vi "USRP Sampling.vi"() -> ()   [LabVIEW 2014]
uses:
  <instrlib>/niUSRP/niUSRP Fetch Rx Data (CDB Cluster).vi
panel:
  out "n":i32
  out "output":dbl[][](array[numeric])
  out "Waveform Graph":dbl[](graph)
  out "Iteration":i32
  out "Array":dbl[](array[numeric])
  in  "stop":bool
  in  "Tab Control":enum32{"USRP Setup", "Parameter"}(tab)
  in  "device names":refnum<k15>="192.168.10.2"
  in  "IQ rate":dbl=800000.0 format="%#_6p"
  in  "carrier frequency":dbl=2422000000.0 format="%#_6p"
  in  "gain":dbl=10.0 format="%#_6f"
  out "coerced IQ rate":dbl=800000.0 format="%#_6p"
  out "coerced carrier frequency":dbl=2421999999.997206 format="%#_6p"
  out "coerced gain":dbl=10.0 format="%#_6f"
  out "error out":errorcluster
  in  "active antenna":string="RX2"
  out "Duration(s)":dbl
  in  "Moving\nAverage":bool=TRUE
  in  "Time Window(s)":dbl=0.01 format="%#_6p"
  in  "SamplingTimes":i32=100
  in  "threshold":dbl=1.0
  in  "step":dbl=1.0
  in  "offset":i32
  in  "Method":enum16{"Binary", "Uniform"}(ring)
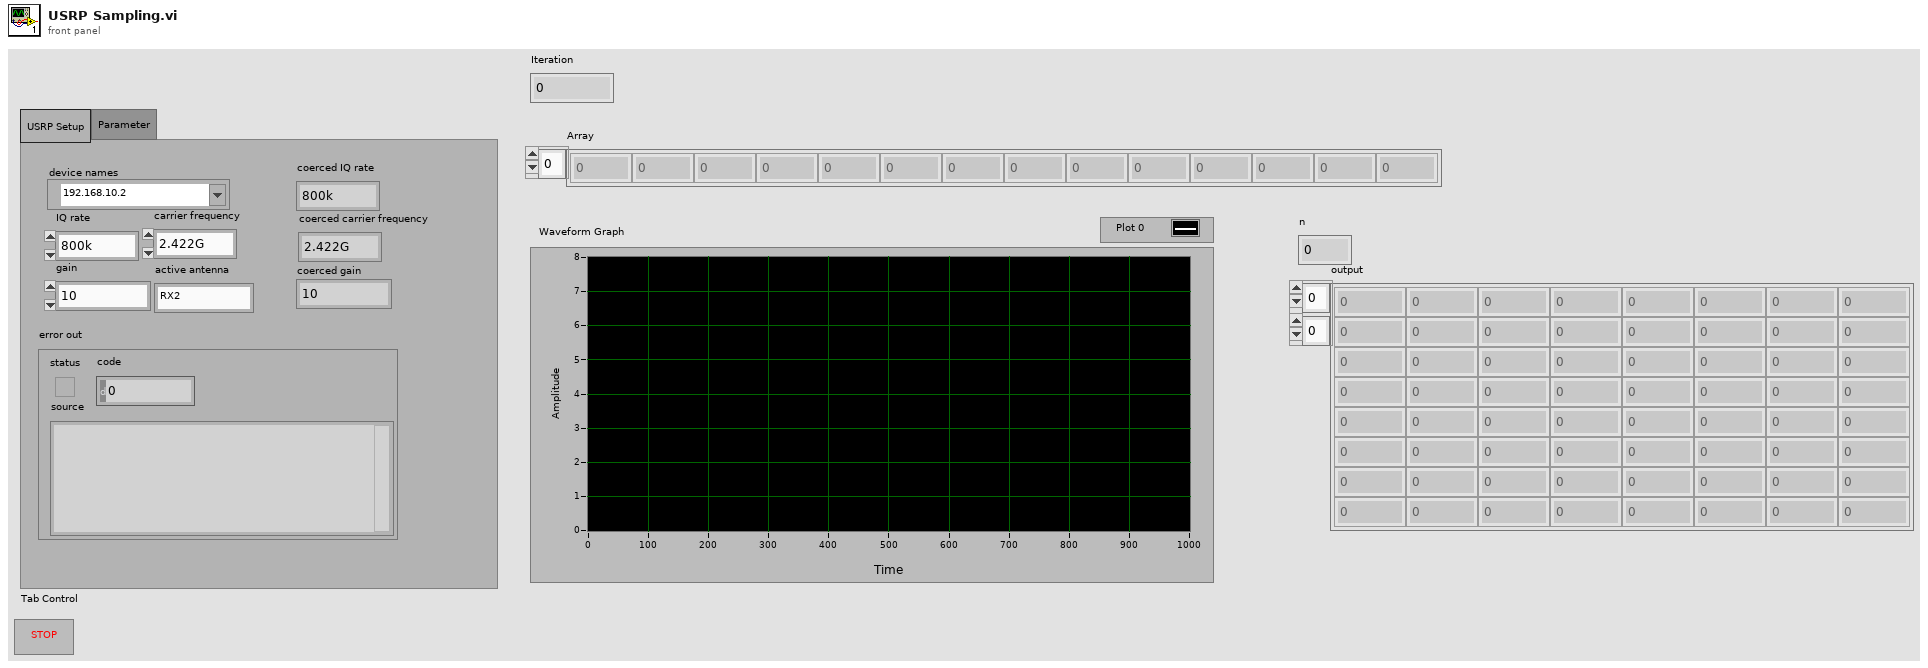
[diagram p1: front panel]
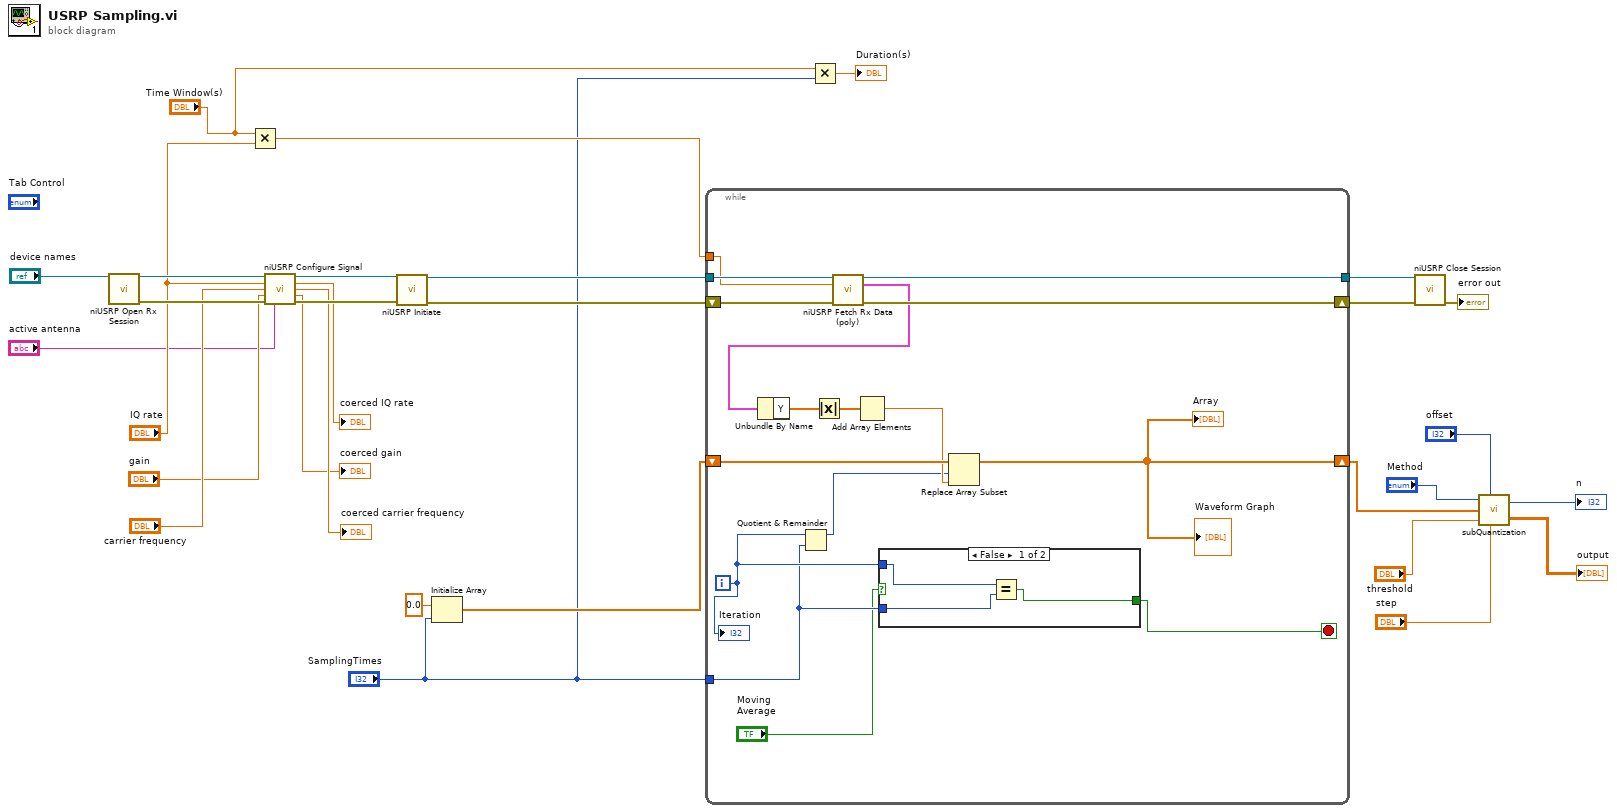
[diagram p0: block diagram]
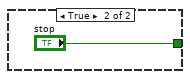
[diagram p2: hidden frame]
diagram:
  n1 = call <instrlib>:"niUSRP Open Rx Session.vi"("device names"="device names") -> ("session handle out"=w28:refnum<k15>, "error out"=w29:errorcluster)  [unwired: 13 in]
  n2 = Multiply(x="Time Window(s)", y="IQ rate") -> (x*y=w11:dbl)
  n3 = call <instrlib>:"niUSRP Configure Signal.vi"("session handle"=w28, "IQ rate"="IQ rate", "carrier frequency"="carrier frequency", "gain"="gain", "error in (no error)"=w29, "active antenna"="active antenna") -> ("session handle out"=w27:refnum<k15>, "coerced IQ rate"=→"coerced IQ rate":dbl, "coerced carrier frequency"=→"coerced carrier frequency":dbl, "coerced gain"=→"coerced gain":dbl, "error out"=w26:errorcluster)  [unwired: 5 in]
  n4 = call <instrlib>:"niUSRP Initiate.vi"("session handle"=w27, "error in (no error)"=w26) -> ("session handle out"=w20:refnum<k15>, "error out"=w19:errorcluster)  [unwired: 12 in]
  n5 = Initialize Array(0.0 ("element"), "SamplingTimes") -> (w13:dbl[])
  n6 = while {
    tunnel: w20 -> [w46]
    tunnel: [w43] -> w17
    shift-right: [w44] -> w18
    shift-left: w19 -> [w45]
    shift-right: [w34] -> w4
    shift-left: w13 -> [w39]
    tunnel: "SamplingTimes" -> [w33]
    tunnel: w11 -> [w32]
    i -> [w35]
    stop <- w36 stop-if-true
    n7 = Quotient & Remainder(x=w35, y=w33) -> (x-y*floor(x/y)=w37:i32)  [unwired: 1 out]
    n8 = call-poly <instrlib>:"niUSRP Fetch Rx Data (poly).vi"("session handle"=w46, "number of samples"=w32, "error in (no error)"=w45) -> ("session handle out"=w43:refnum<k15>, "data"=w42:cluster{"t0":dbl, "dt":dbl, "Y":cdb[]}, "error out"=w44:errorcluster)  [unwired: 9 in, 1 out]
    n9 = Unbundle By Name(w42) -> ("Y"=w41:cdb[])
    n10 = Absolute Value(x=w41) -> (abs(x)=w40:dbl[])
    n11 = Add Array Elements(numeric array=w40) -> (sum=w38:dbl)
    n12 = case shown="False" "Moving\nAverage" {
      tunnel: [w47 "stop"] -> w36
      tunnel: w35 -> [w49 _]
      tunnel: w33 -> [w48 _]
      frame False {
        n13 = Equal?(x=w49, y=w48) -> (x = y?=w47:bool)
      }
      frame True {
      }
    }
    n14 = Replace Array Subset(array=w39, new element=w38, index=w37) -> (w34:dbl[])
    "Array" <- w34
    "Waveform Graph" <- w34
    "Iteration" <- w35
  }
  n15 = Multiply(x="Time Window(s)", y="SamplingTimes") -> (x*y=→"Duration(s)":dbl)
  n16 = call <instrlib>:"niUSRP Close Session.vi"("session handle"=w17, "error in (no error)"=w18) -> ("error out"=→"error out":errorcluster)  [unwired: 13 in]
  n17 = call "subQuantization.vi"("Method"="Method", "offset"="offset", "input"=w4, "threshold"="threshold", "step"="step") -> ("n"=→"n":i32, "output"=→"output":dbl[][])
